vi "WSVCAP SHL FPGA LL Procedure I2C - Send Address Byte.vi"(0 "Procedure Step":T1, 1 "Wait Ticks Remaining":u32, 5 "I2C Wait Ticks":u32, 7 "Write Bits Remaining":u8, 9 "Write Byte":u8, 11 "error in (no error)":errorcluster, 13 "Socket Mask":u64 format="%012x") -> (3 "Wait Ticks Remaining Out":u32, 4 "Procedure Step Out":T1, 8 "Write Bits Remaining Out":u8, 10 "Finished":bool, 15 "error out":errorcluster)   [LabVIEW 2012]
uses:
  Type Defs/WSVCAP SHL Procedure Step Enum.ctl
  Type Defs/WSVCAP SHL I2C Write Line Enum.ctl
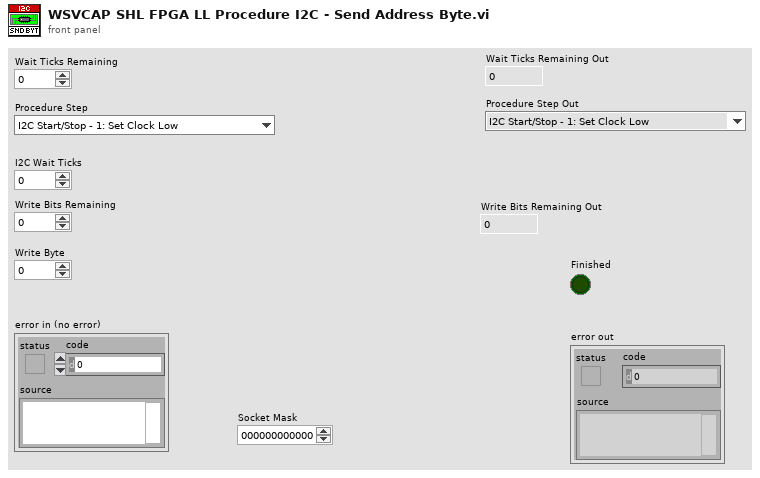
[diagram p1: front panel]
types:
  T1 = typedef "WSVCAP SHL Procedure Step Enum.ctl" = enum16{"I2C Start/Stop - 1: Set Clock Low", "I2C Start/Stop - 2: Wait", "I2C Start/Stop - 3: Set Data I", "I2C Start/Stop - 4: Wait", "I2C Start/Stop - 5: Set Clock High", "I2C Start/Stop - 6: Wait", "I2C Start/Stop - 7: Set Data II", "I2C Start/Stop - 8: Wait", "I2C Start/Stop - 9: Set Clock Low", "I2C Start/Stop - 10: Wait", "I2C Read ACK - 1: Set Clock High", "I2C Read ACK - 2: Wait", "I2C Read ACK - 3: Read ACK Bit", "I2C Read ACK - 4: Wait", "I2C Read ACK - 5: Set Clock Low", "I2C Read ACK - 6: Wait", "I2C Write ACK - 1: Write ACK Bit", "I2C Write ACK - 2: Wait", "I2C Write ACK - 3: Set Clock High", "I2C Write ACK - 4: Wait", "I2C Write ACK - 5: Set Clock Low", "I2C Write ACK - 6: Wait", "I2C Write ACK - 7: Set Data Low", "I2C Send Add - 1: Reset Bits Remaining", "I2C Send Add - 2: Set Data Bit", "I2C Send Add - 3: Wait", "I2C Send Add - 4: Set Clock High", "I2C Send Add - 5: Wait", "I2C Send Add - 6: Set Clock Low", "I2C Send Add - 7: Wait", "I2C Send Add - 8: Check Bits Remaining", "I2C Send Data - 1: Reset Bits Remaining", "I2C Send Data - 2: Load Write Bit from FIFO", "I2C Send Data - 3: Set Data Bit", "I2C Send Data - 4: Wait", "I2C Send Data - 5: Set Clock High", "I2C Send Data - 6: Wait", "I2C Send Data - 7: Set Clock Low", "I2C Send Data - 8: Wait", "I2C Send Data - 9: Check Bits Remaining", "I2C Receive Data - 1: Reset Bits Remaining", "I2C Receive Data - 2: Wait", "I2C Receive Data - 3: Set Clock High", "I2C Receive Data - 4: Wait", "I2C Receive Data - 5: Read Data Bit", "I2C Receive Data - 6: Wait", "I2C Receive Data - 7: Set Clock Low", "I2C Receive Data - 8: Wait", "I2C Receive Data - 9: Check Bits Remaining", "SPI Clear Lines - 1:Clear", "SPI Send/Receive - 1: Load SDA - Clock Low", "SPI Send/Receive - 2: Wait", "SPI Send/Receive - 3: Load DATO - Clock High", "SPI Send/Receive - 4: Wait", "SPI Wait CMD Delay - 1:Wait", "RFFE Send SSC - 1:Set Low", "RFFE Send SSC - 2:Wait", "RFFE Send SSC - 3:Set SDA High", "RFFE Send SSC - 4:Wait", "RFFE Send SSC - 5:Set SDA Low", "RFFE Send SSC - 6:Wait", "RFFE Send Data - 1:Set SCL High", "RFFE Send Data - 2:Wait", "RFFE Send Data - 3:Set SCL Low", "RFFE Send Data - 4:Wait", "RFFE Send Data - 5:Set SCL High (P)", "RFFE Send Data - 6:Wait", "RFFE Send Data - 7:Set SCL Low (P)", "RFFE Send Data - 8:Wait", "RFFE Send Data - 9:Set SCL High (BP)", "RFFE Send Data - 10:Wait", "RFFE Send Data - 11:Set SCL Low (BP)", "RFFE Send Data - 12:Wait", "RFFE Receive Data - 1:Set SCL High", "RFFE Receive Data - 2:Wait", "RFFE Receive Data - 3:Set SCL Low", "RFFE Receive Data - 4:Wait", "RFFE Receive Data - 5:Set SCL High (BP)", "RFFE Receive Data - 6:Wait", "RFFE Receive Data - 7:Set SCL Low (BP)", "RFFE Receive Data - 8:Wait", "RFFE Wait CMD Delay - 1:Wait", "RFFE Clear Lines - 1:Clear"}
  T2 = typedef "WSVCAP SHL I2C Write Line Enum.ctl" = enum16{"I2C SCL", "I2C SDA"}
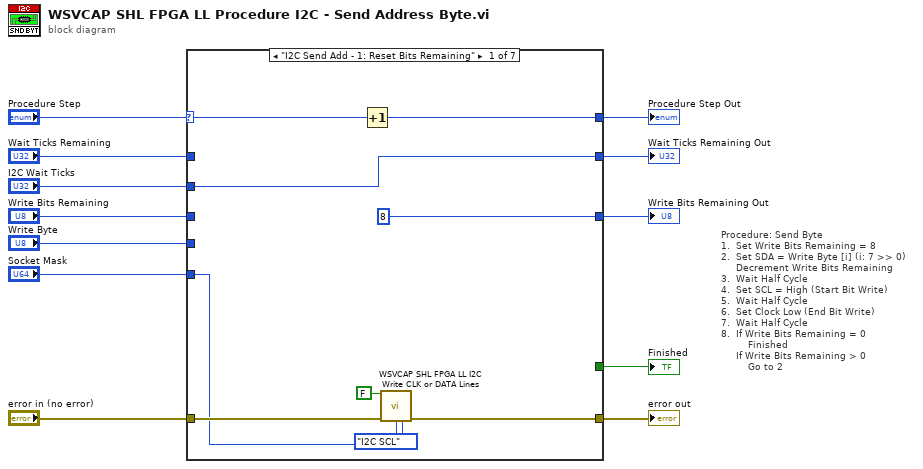
[diagram p0: block diagram]
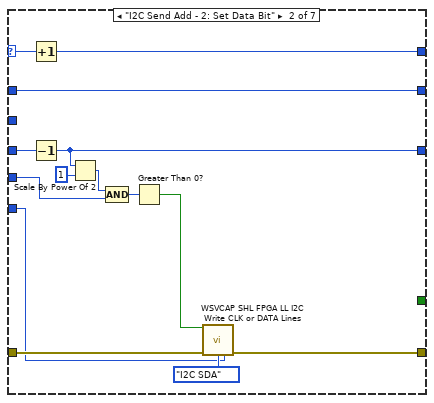
[diagram p2: hidden frame]
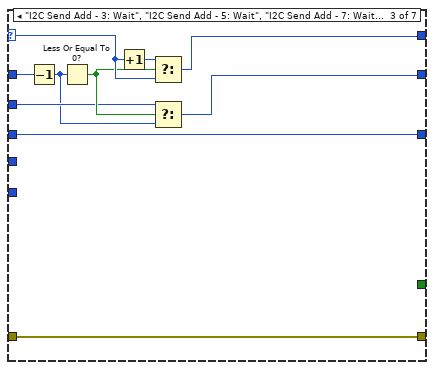
[diagram p3: hidden frame]
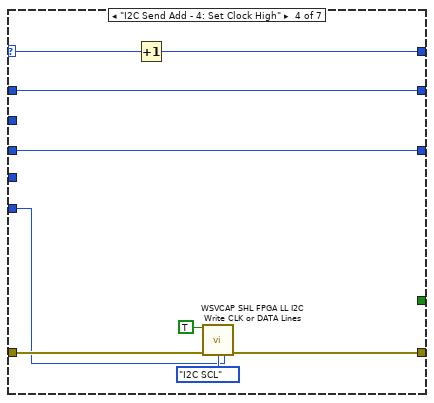
[diagram p4: hidden frame]
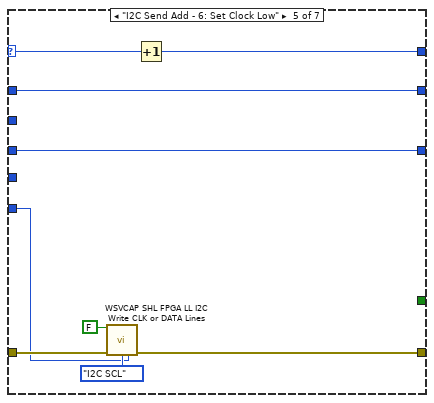
[diagram p5: hidden frame]
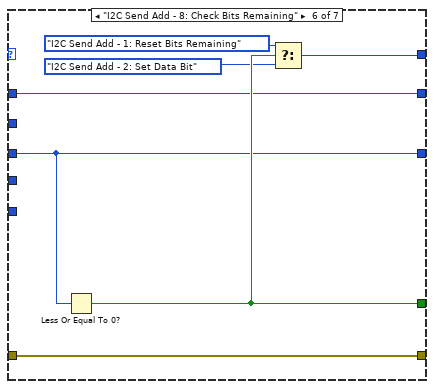
[diagram p6: hidden frame]
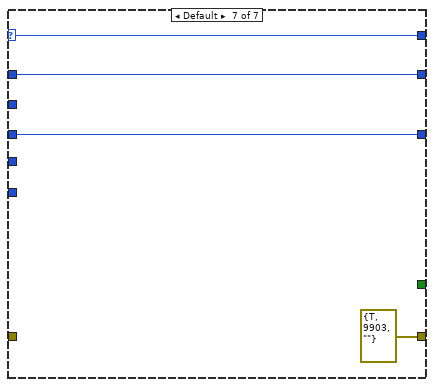
[diagram p7: hidden frame]
diagram:
  # "Procedure: Send Byte\n1.  Set Write Bits Remaining = 8\n2.  Set SDA = Write Byte [i] (i: 7 >> 0)\n     Decrement Write Bits Remaining\n3.  Wait Half Cycle\n4.  Set SCL = High (Start Bit Write)\n5.  Wait Half Cycle\n6.  Set Clock Low (End Bit Write)\n7.  Wait Half Cycle\n8.  If Write Bits Remaining = 0\n         Finished\n     If Write Bits Remaining > 0\n         Go to 2"
  n1 = case shown="\"I2C Send Add - 1: Reset Bits Remaining\"" "Procedure Step" {
    selector: "Procedure Step" -> [w17 w32 w44 w51 w59 _ w73]
    tunnel: [w19 w33 w42 w52 w61 w70 errorcluster {"status"=TRUE, "code"=9903, "source"=""} ("error IO")] -> w11
    tunnel: "error in (no error)" -> [w20 w34 w42 w53 w62 w70 _]
    tunnel: "Wait Ticks Remaining" -> [_ w22 w45 w47 w56 w64 w72]
    tunnel: "I2C Wait Ticks" -> [w13 _ w40 _ _ _ _]
    tunnel: "Write Bits Remaining" -> [_ w27 w36 w46 w55 w65 w71]
    tunnel: "Write Byte" -> [_ w26 _ _ _ _ _]
    tunnel: [_ _ _ _ _ w69 _] -> w10
    tunnel: "Socket Mask" -> [w16 w25 _ w49 w58 _ _]
    tunnel: [w15 w24 w38 w48 w57 w66 w73] -> w3
    tunnel: [w13 w22 w37 w47 w56 w64 w72] -> w2
    tunnel: [u8 8 ("Write Bits Remaining") w23 w36 w46 w55 w65 w71] -> w1
    frame "I2C Send Add - 1: Reset Bits Remaining" {
      n2 = Increment(x=w17) -> (x+1=w15:T1)
      n3 = call "WSVCAP SHL FPGA LL I2C Write CLK or DATA Lines.vi"("Bit In"=FALSE, "error in (no error)"=w20, "Line"=WSVCAP_SHL_I2C_Write_Line_Enum."I2C SCL", "Socket Mask"=w16) -> ("error out"=w19:errorcluster)  [unwired: 11 in]
    }
    frame "I2C Send Add - 2: Set Data Bit" {
      n4 = Increment(x=w32) -> (x+1=w24:T1)
      n5 = Decrement(x=w27) -> (x-1=w23:u8)
      n6 = Scale By Power Of 2(n=w23, x=u8 1 ("Write Bits Remaining")) -> (x*2^n=w30:u8)
      n7 = Compound Arithmetic op=AND(w30, w26) -> (w29:u8)
      n8 = Greater Than 0?(x=w29) -> (x > 0?=w28:bool)
      n9 = call "WSVCAP SHL FPGA LL I2C Write CLK or DATA Lines.vi"("Bit In"=w28, "error in (no error)"=w34, "Line"=WSVCAP_SHL_I2C_Write_Line_Enum."I2C SDA", "Socket Mask"=w25) -> ("error out"=w33:errorcluster)  [unwired: 11 in]
    }
    frame "I2C Send Add - 3: Wait", "I2C Send Add - 5: Wait", "I2C Send Add - 7: Wait" {
      n10 = Decrement(x=w45) -> (x-1=w39:u32)
      n11 = Less Or Equal To 0?(x=w39) -> (x <= 0?=w41:bool)
      n12 = Increment(x=w44) -> (x+1=w43:T1)
      n13 = Select(t=w43, s=w41, f=w44) -> (s? t:f=w38:T1)
      n14 = Select(t=w40, s=w41, f=w39) -> (s? t:f=w37:u32)
    }
    frame "I2C Send Add - 4: Set Clock High" {
      n15 = Increment(x=w51) -> (x+1=w48:T1)
      n16 = call "WSVCAP SHL FPGA LL I2C Write CLK or DATA Lines.vi"("Bit In"=TRUE, "error in (no error)"=w53, "Line"=WSVCAP_SHL_I2C_Write_Line_Enum."I2C SCL", "Socket Mask"=w49) -> ("error out"=w52:errorcluster)  [unwired: 11 in]
    }
    frame "I2C Send Add - 6: Set Clock Low" {
      n17 = call "WSVCAP SHL FPGA LL I2C Write CLK or DATA Lines.vi"("Bit In"=FALSE, "error in (no error)"=w62, "Line"=WSVCAP_SHL_I2C_Write_Line_Enum."I2C SCL", "Socket Mask"=w58) -> ("error out"=w61:errorcluster)  [unwired: 11 in]
      n18 = Increment(x=w59) -> (x+1=w57:T1)
    }
    frame "I2C Send Add - 8: Check Bits Remaining" {
      n19 = Less Or Equal To 0?(x=w65) -> (x <= 0?=w69:bool)
      n20 = Select(t=WSVCAP_SHL_Procedure_Step_Enum."I2C Send Add - 1: Reset Bits Remaining" ("Procedure Step"), s=w69, f=WSVCAP_SHL_Procedure_Step_Enum."I2C Send Add - 2: Set Data Bit" ("Procedure Step")) -> (s? t:f=w66:T1)
    }
    frame Default {
    }
  }
  "error out" <- w11
  "Finished" <- w10
  "Procedure Step Out" <- w3
  "Wait Ticks Remaining Out" <- w2
  "Write Bits Remaining Out" <- w1
